vi "Check Method Server Streaming.vi"(8 "error in (no error)":errorcluster, 11 "Method ref in":u64) -> (0 "error out":errorcluster, 2 "is Server Streaming":bool, 3 "Method ref out":u64)   [LabVIEW 2019, in "gRPC Scripting Tools.lvlib"]
uses:
  gRPC Scripting Tools.lvlib
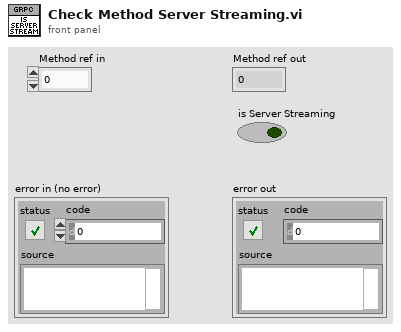
[diagram p1: front panel]
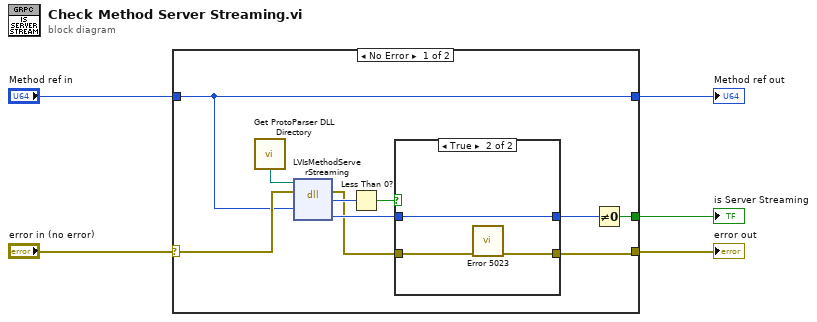
[diagram p0: block diagram]
diagram:
  n1 = case shown="No Error" "error in (no error)" {
    selector: "error in (no error)" -> [w13 w21]
    tunnel: [w15 _] -> w5
    tunnel: "Method ref in" -> [w12 w22]
    tunnel: [w12 w22] -> w2
    tunnel: [w9 w21] -> w1
    frame No Error {
      n2 = call "Get ProtoParser DLL Directory.vi"() -> ("Proto Parser Directory"=w14:path)
      n3 = dll-call lib="C:/Users/XEnderMD/Desktop/LV gRPC/labview source/gRPC Scripting Tools/Proto Parser API/dll/labview_grpc_generator.dll" fn="LVIsMethodServerStreaming"(path in=w14, error in=w13, "method"=w12) -> (error out=w6:errorcluster, "return type"=w11:i32, "serverStreaming"=w8:i32)  [unwired: 3 in, 1 out]
      n4 = Less Than 0?(x=w11) -> (x < 0?=w10:bool)
      n5 = case shown="True" w10 {
        tunnel: [w17 w20] -> w9
        tunnel: w8 -> [w16 w19]
        tunnel: [w16 w19] -> w7
        tunnel: w6 -> [w17 w18]
        frame False {
        }
        frame True {
          n6 = call "Error 5023.vi"("error in (no error)"=w18) -> ("error out"=w20:errorcluster)  [unwired: 10 in]
        }
      }
      n7 = Not Equal To 0?(x=w7) -> (x != 0?=w15:bool)
    }
    frame Error {
    }
  }
  "is Server Streaming" <- w5
  "Method ref out" <- w2
  "error out" <- w1
